vi "Unregister Broadcast.vi"(0 "CSM Name":string, 1 "TcpRouter-Client in":refnum<class "TcpRouter-Client.lvclass">, 5 "Source CSM Name (* as Default)":string="*", 7 "Status":string, 9 "Response Message (if \"\", same as Source Message)":string, 11 "error in (no error)":errorcluster, 12 "Response Timeout(5000ms)":i32=5000) -> (4 "CSM Name(dup)":string, 15 "error out":errorcluster)   [LabVIEW 2020, in "CSM-TCP-Router.lvlib" / "TcpRouter-Client.lvclass"]
uses:
  TcpRouter-Client.lvclass
  TcpRouter-Client.lvclass/TcpRouter-Client.ctl
  _support/tcp-msg type.ctl
  f32241c3-0036-4787-bc41-e9c1f987f5e1.vi
  <userlib>/_NEVSTOP/Communicable State Machine(CSM)/AdvanceAPI/CSM - Revert Arguments-Safe String.vi
  <userlib>/_NEVSTOP/Communicable State Machine(CSM)/_Shared/Trim Single-line Text.vi
  <userlib>/_NEVSTOP/Communicable State Machine(CSM)/AdvanceAPI/CSM - Keywords.vi
  <userlib>/_NEVSTOP/Communicable State Machine(CSM)/_Polymophic/Build Unregister Message.vi
  CSM-TCP-Router.lvlib
  <userlib>/_NEVSTOP/Communicable State Machine(CSM)/Communicable State Machine.lvlib
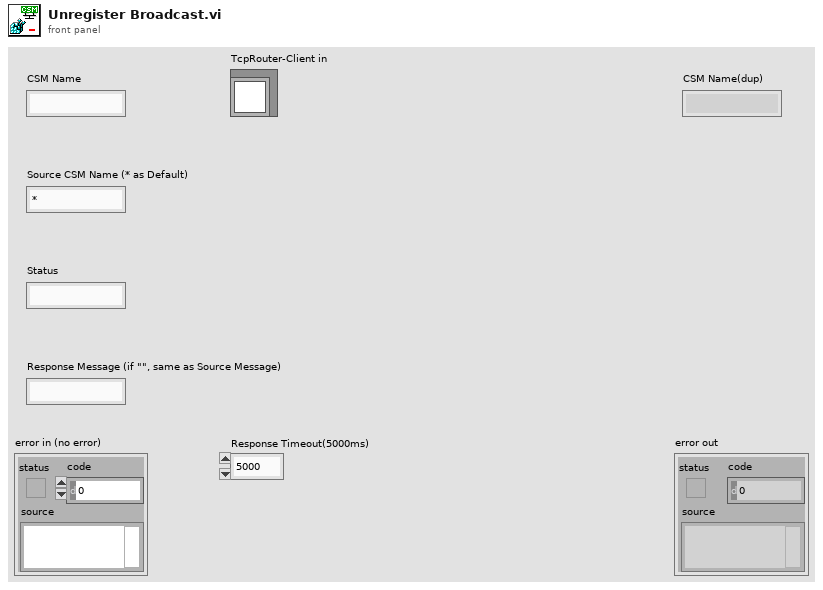
[diagram p1: front panel]
types:
  T1 = typedef "CSM-TCP-Router.lvlib/tcp-msg type.ctl" = enum8{"info", "error", "cmd", "cmd-resp", "resp", "async-resp", "status", "interrupt"}
  T2 = typedef "CSM-TCP-Router.lvlib/TcpRouter-Client.lvclass/Def-TCP-Router REQ-REP.ctl" = cluster{"REQ-REP":refnum<k5>}
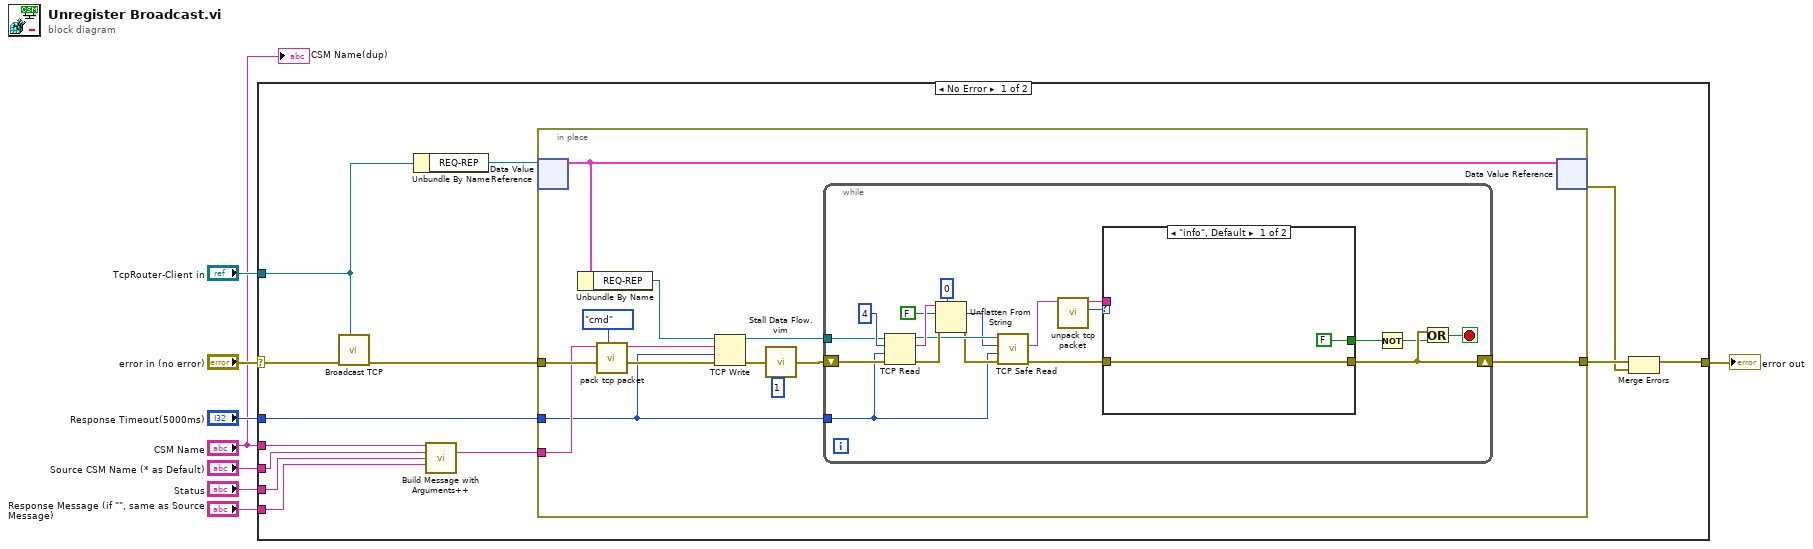
[diagram p0: block diagram]
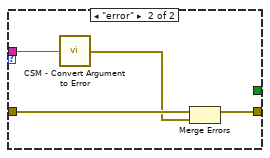
[diagram p2: hidden frame]
diagram:
  n1 = case shown="No Error" "error in (no error)" {
    selector: "error in (no error)" -> [w21 w59]
    tunnel: [w10 w59] -> w7
    tunnel: "TcpRouter-Client in" -> [w12 _]
    tunnel: "Response Timeout(5000ms)" -> [w17 _]
    tunnel: "CSM Name" -> [w16 _]
    tunnel: "Source CSM Name (* as Default)" -> [w15 _]
    tunnel: "Status" -> [w14 _]
    tunnel: "Response Message (if \"\", same as Source Message)" -> [w13 _]
    frame No Error {
      n2 = call "Broadcast TCP.vi"("TcpRouter-Client in"=w12, "error in (no error)"=w21) -> ("error out"=w20:errorcluster)  [unwired: 8 in, 1 out]
      n3 = Unbundle By Name(w12) -> ("REQ-REP"=w11:refnum<data-value>)
      n4 = call-poly <userlib>:"Build Message with Arguments++.vi"("Target CSM"=w16, "Source CSM (* as Default)"=w15, "Status"=w14, "API (* as Default)"=w13) -> ("CSM Message String"=w19:string)  [unwired: 11 in]
      n5 = in-place {
        in-place-border: w20 -> [w31]
        in-place-border: w19 -> [w30]
        in-place-border: [w25] -> w18
        in-place-border: w17 -> [w24]
        n6 = in-place-dvr #1(w11) -> (w23:T2)  [unwired: 1 out]
        n7 = Unbundle By Name(w23) -> ("REQ-REP"=w22:refnum<k5>)
        n8 = call "pack tcp packet.vi"("tcp-message-type"=tcp-msg_type."cmd", "String"=w30) -> ("TCP Pack"=w33:string)  [unwired: 9 in]
        n9 = TCP Write(connection ID=w22, data in=w33, error in (no error)=w31, 9:w24) -> (connection ID out=w27:refnum<k5>, error out=w29:errorcluster)  [unwired: 1 out]
        n10 = call "Stall Data Flow.vim"("value in"=w29, "milliseconds to wait"=u32 1) -> ("value out"=w26:errorcluster)  [unwired: 1 out]
        n11 = while {
          tunnel: w27 -> [w43]
          shift-right: [w38] -> w25
          shift-left: w26 -> [w42]
          tunnel: w24 -> [w37]
          stop <- w36 stop-if-true
          n12 = TCP Read(connection ID=w43, bytes to read=4, error in (no error)=w42, 9:w37) -> (connection ID out=w50:refnum<k5>, data out=w51:string, error out=w52:errorcluster)  [unwired: 1 in]
          n13 = Unflatten From String(type=0, binary string=w51, data includes array or string size? (T)=FALSE, error in (no error)=w52) -> (value=w48:i32, error out=w47:errorcluster)  [unwired: 2 out]
          n14 = call "TCP Safe Read.vi"("error in (no error)"=w47, "timeout ms (25000)"=w37, "bytes to read"=w48, "TCP Network Connection in"=w50) -> ("error out"=w40:errorcluster, "String"=w49:string)  [unwired: 5 in, 1 out]
          n15 = call "unpack tcp packet.vi"("TCP Pack"=w49) -> ("tcp-message-type"=w41:T1, "String"=w39:string)  [unwired: 9 in]
          n16 = case shown="\"info\", Default" w41 {
            tunnel: w40 -> [w54 w58]
            tunnel: [w54 w56] -> w38
            tunnel: w39 -> [_ w57]
            tunnel: [FALSE _] -> w35
            frame "info", Default {
            }
            frame "error" {
              n17 = call <userlib>:"CSM - Convert Argument to Error.vi"("Argument"=w57) -> ("Error"=w55:errorcluster)  [unwired: 4 in]
              n18 = Merge Errors(w58, w55) -> (w56:errorcluster)
            }
          }
          n19 = Not(x=w35) -> (.not. x?=w34:bool)
          n20 = Or(x=w38, y=w34) -> (x .or. y?=w36:bool)
        }
        n21 = in-place-dvr #1(w23) -> (w9:errorcluster)  [unwired: 1 out]
      }
      n22 = Merge Errors(w18, w9) -> (w10:errorcluster)
    }
    frame Error {
    }
  }
  "error out" <- w7
  "CSM Name(dup)" <- "CSM Name"
